vi "GET.series.by_id.vi"(5 "request specific headers":T2[](array[typedef]), 7 "timeout (60000)":i32=60000, 8 "error in (no error)":errorcluster, 10 "id":string, 11 "REST Client in":refnum<class "REST Client.lvclass">) -> (0 "error out":errorcluster, 2 "data":T1, 3 "REST Client out":refnum<class "REST Client.lvclass">)   [LabVIEW 2024]
uses:
  <vilib>/addons/_JKI.lib/REST Client/classes/REST Client/HTTP Header.ctl
  <vilib>/NI/Advanced HTTP Client/Header--Combo Box.ctl
  <vilib>/addons/_JKI.lib/REST Client/classes/REST Client/REST Client.lvclass
  TypeDefs/series.reply.ctl
  <vilib>/NI/Advanced HTTP Client/Session.lvclass
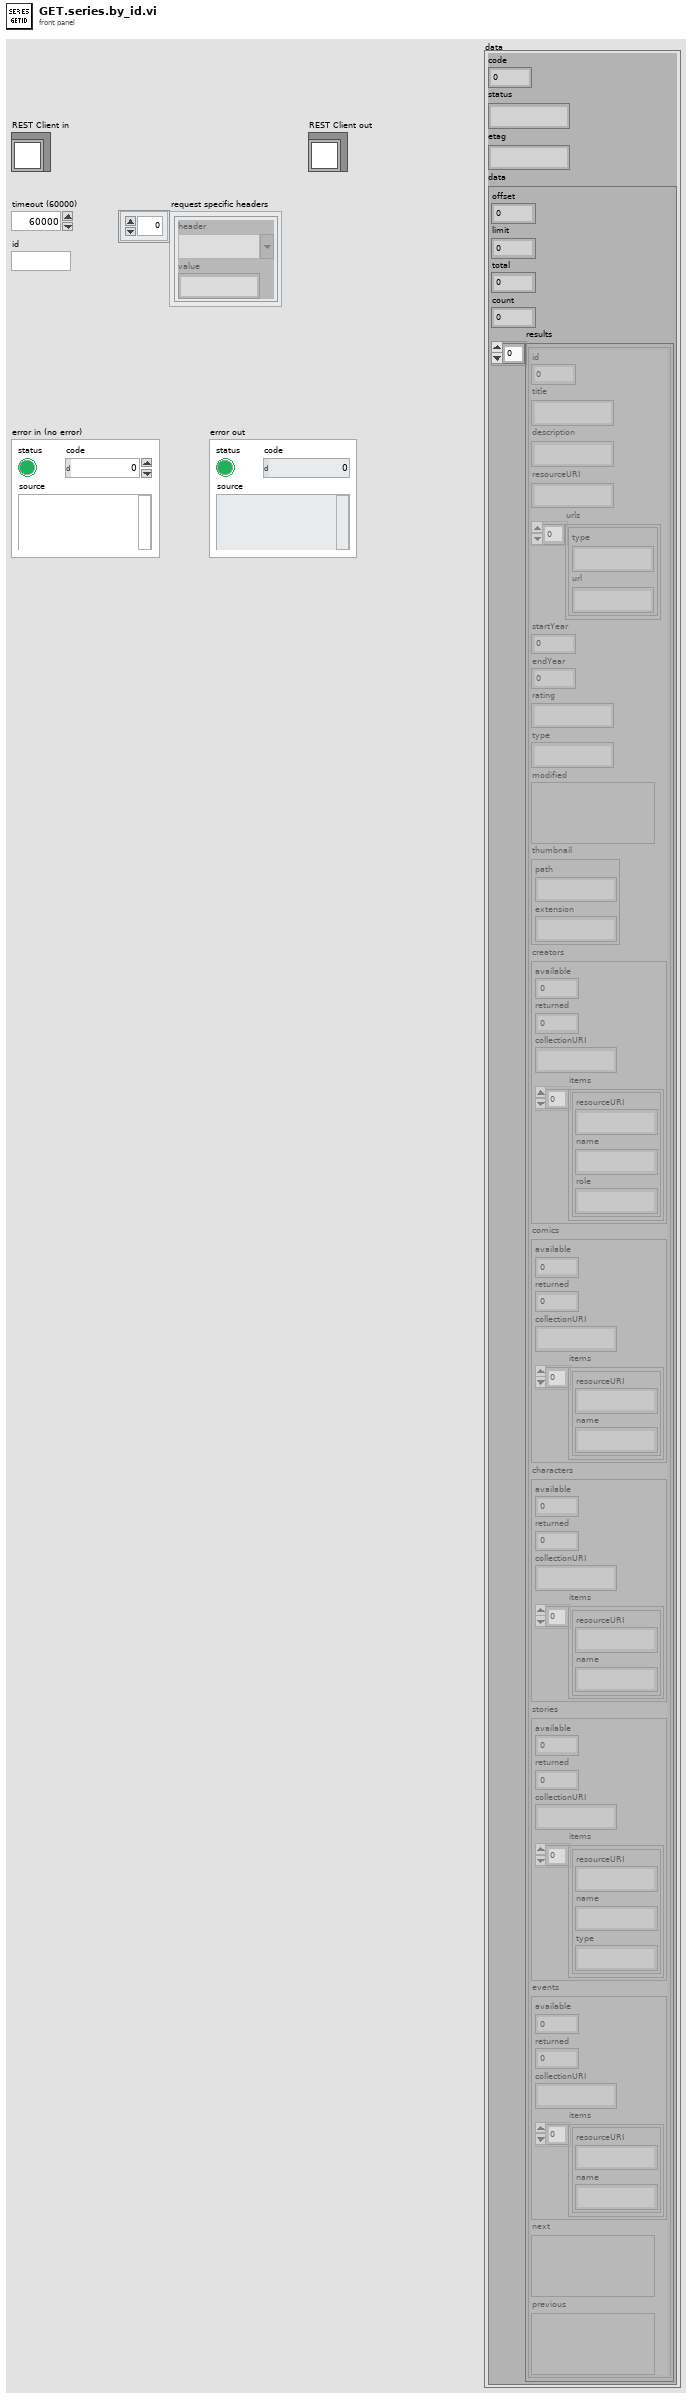
[diagram p1: front panel]
types:
  T1 = typedef "series.reply.ctl" = cluster{"code":i32, "status":string, "etag":string, "data":cluster{"offset":i32, "limit":i32, "total":i32, "count":i32, "results":cluster{"id":i32, "title":string, "description":string, "resourceURI":string, "urls":cluster{"type":string, "url":string}[], "startYear":i32, "endYear":i32, "rating":string, "type":string, "modified":variant, "thumbnail":cluster{"path":string, "extension":string}, "creators":cluster{"available":i32, "returned":i32, "collectionURI":string, "items":cluster{"resourceURI":string, "name":string, "role":string}[]}, "comics":cluster{"available":i32, "returned":i32, "collectionURI":string, "items":cluster{"resourceURI":string, "name":string}[]}, "characters":cluster{"available":i32, "returned":i32, "collectionURI":string, "items":cluster{"resourceURI":string, "name":string}[]}, "stories":cluster{"available":i32, "returned":i32, "collectionURI":string, "items":cluster{"resourceURI":string, "name":string, "type":string}[]}, "events":cluster{"available":i32, "returned":i32, "collectionURI":string, "items":cluster{"resourceURI":string, "name":string}[]}, "next":variant, "previous":variant}[]}}
  T2 = typedef "REST Client.lvlib/REST Client.lvclass/HTTP Header.ctl" = cluster{"header":T3, "value":string}
  T3 = typedef "lib_NI_Advanced HTTP Client.lvlib/Session.lvclass/Header--Combo Box.ctl" = string
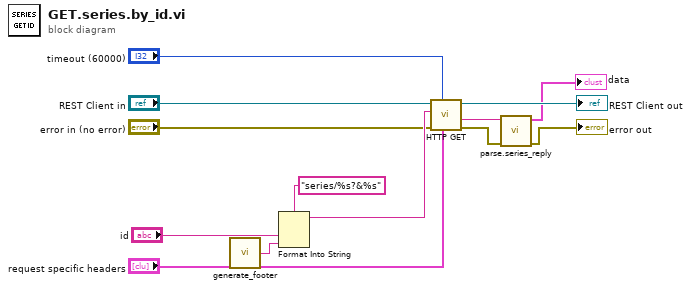
[diagram p0: block diagram]
diagram:
  n1 = call "generate_footer.vi"() -> ("footer"=w8:string)  [unwired: 1 in]
  n2 = Format Into String(format string="series/%s?&%s" ("Path"), "id", w8) -> (resulting string=w9:string)  [unwired: 2 in, 1 out]
  n3 = call-dynamic "HTTP GET.vi"("request specific headers"="request specific headers", "timeout (0 = Use Default)"="timeout (60000)", "error in (no error)"="error in (no error)", "Path"=w9, "REST Client in"="REST Client in") -> ("error out"=w11:errorcluster, "Response body"=w10:string, "REST Client out"=→"REST Client out":refnum<class "REST Client.lvclass">)  [unwired: 1 in, 3 out]
  n4 = call "parse.series_reply.vi"("error in"=w11, "string in"=w10) -> ("error out"=→"error out":errorcluster, "data"=→"data":T1)  [unwired: 8 in]
